vi "Get Camera Names.vi"(8 "error IO":errorcluster, 11 "Default JSON in":variant) -> (0 "error out":errorcluster, 3 "Camera Names":string[](array[string]))   [LabVIEW 2015, in "ZenGage v3.0 UI.lvclass"]
uses:
  ZenGage v3.0 UI.lvclass
  Common/Controls/ImageAcquisitionParameters.ctl
panel:
  out "Error Message":string
  out "VCluster\n out":variant
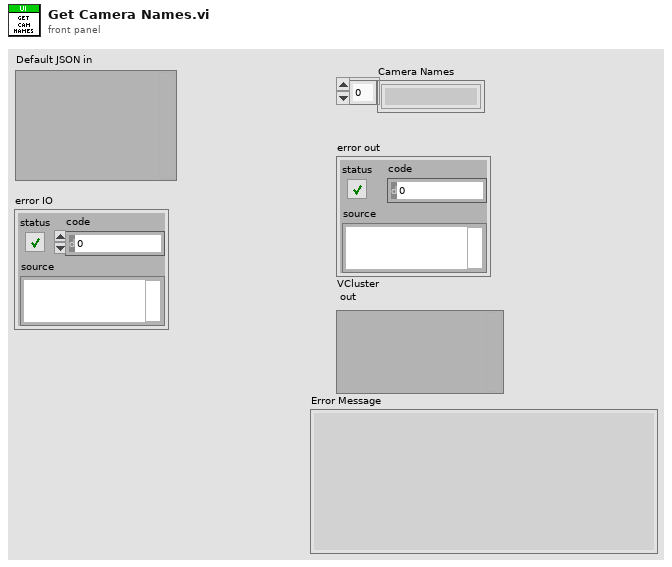
[diagram p1: front panel]
types:
  T1 = typedef "ImageAcquisitionParameters.ctl" = cluster{"ImageAcquisitionParameters":cluster{"Id":dbl, "SessionID":string, "Type":string, "Model":string, "InterfaceType":string, "SerialNumber":string, "Timeout":dbl, "GeneralCameraConfig":cluster{"ActiveAttribute":string, "Value":string}[], "DefaultAOI":i32[], "DefaultReceiverSequence":cluster{"ReceiverID":dbl, "Index":dbl}[], "DefaultfileName":string, "Continuous":dbl, "NumberOfBuffers":dbl, "BufferNumberMode":dbl, "acquisitionTimeout":dbl, "ImageType":dbl, "Offline":bool, "ColorCameraParam":cluster{"PixelFormat":string, "GammaEnable":bool, "GammaSelector":string, "BalanceRationSelector":string[], "BalanceRationRaw":i32[], "BalanceWhiteAuto":string, "LightSourceSelector":string}, "PartsList":cluster{"Name":string, "ReceiverSequence":cluster{"ReceiverID":dbl, "Index":dbl}[], "AOI":i32[], "filePath":string}[]}[]}
  T2 = cluster{"Id":dbl, "SessionID":string, "Type":string, "Model":string, "InterfaceType":string, "SerialNumber":string, "Timeout":dbl, "GeneralCameraConfig":cluster{"ActiveAttribute":string, "Value":string}[], "DefaultAOI":i32[], "DefaultReceiverSequence":cluster{"ReceiverID":dbl, "Index":dbl}[], "DefaultfileName":string, "Continuous":dbl, "NumberOfBuffers":dbl, "BufferNumberMode":dbl, "acquisitionTimeout":dbl, "ImageType":dbl, "Offline":bool, "ColorCameraParam":cluster{"PixelFormat":string, "GammaEnable":bool, "GammaSelector":string, "BalanceRationSelector":string[], "BalanceRationRaw":i32[], "BalanceWhiteAuto":string, "LightSourceSelector":string}, "PartsList":cluster{"Name":string, "ReceiverSequence":cluster{"ReceiverID":dbl, "Index":dbl}[], "AOI":i32[], "filePath":string}[]}[]
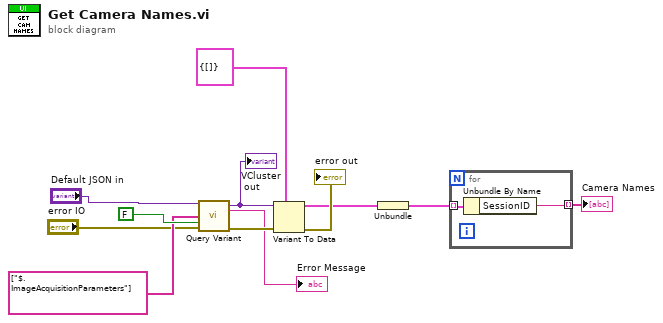
[diagram p0: block diagram]
diagram:
  n1 = call <vilib>:"Query Variant.vi"("VCluster in"="Default JSON in", "pathList"=string[] ["$.ImageAcquisitionParameters"], "Reorder\nqueried\nvariants?"=FALSE ("Reorder\nqueried\nvariants?"), "error IO"="error IO") -> ("VCluster\n out"=w11:variant, "Error Message"=→"Error Message":string, "error out"=w12:errorcluster)  [unwired: 8 in, 1 out]
  "VCluster\n out" <- w11
  n2 = Variant To Data(error in=w12, type=T1 {"ImageAcquisitionParameters"=[]} ("ImageAcquisitionParameters"), Variant=w11) -> (data=w6:T1, error out=→"error out":errorcluster)
  n3 = Unbundle(w6) -> ("ImageAcquisitionParameters"=w5:T2)
  n4 = for {
    tunnel: w5 -> [w14] mode=indexing
    tunnel: [w13] -> w4 mode=indexing
    n5 = Unbundle By Name(w14) -> ("SessionID"=w13:string)
  }
  "Camera Names" <- w4
